vi "LvJDS2900_Sub_Inquiry.vi"(8 "error in (no error)":errorcluster caption="エラー入力（エラーなし）", 10 "Command":string, 11 "VISA rsrc":refnum<visa-resource-name>) -> (0 "error out":errorcluster caption="エラー出力", 1 "Response":string, 3 "VISA rsrc out":refnum<visa-resource-name>)   [LabVIEW 2014]
panel:
  # ":r<nn>=<x>"
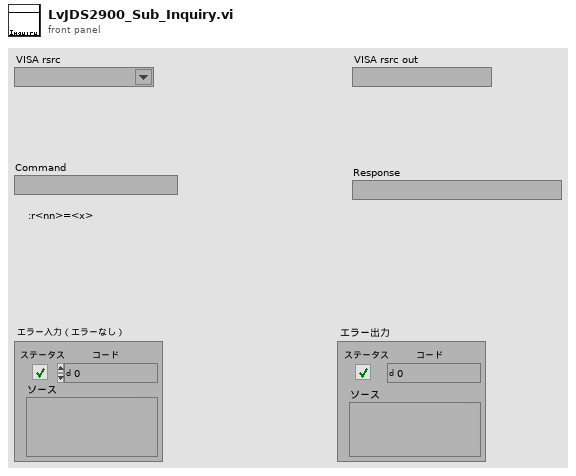
[diagram p1: front panel]
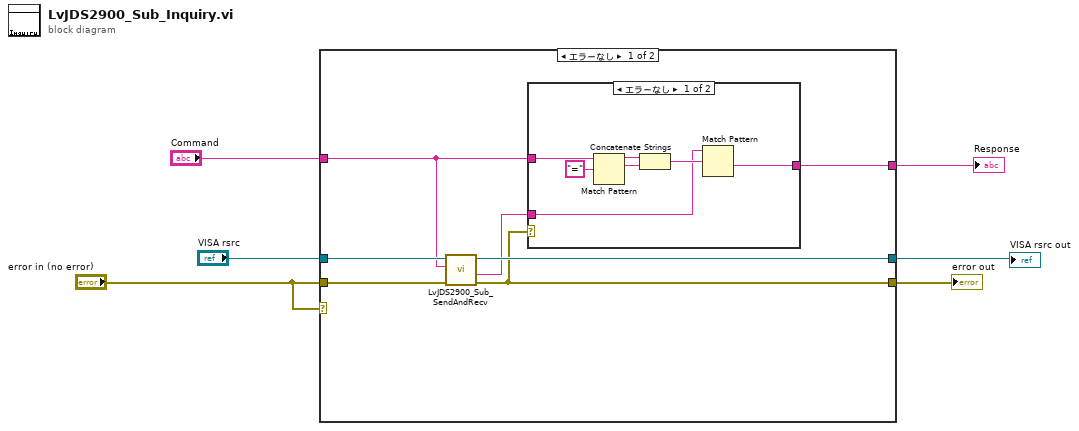
[diagram p0: block diagram]
diagram:
  n1 = case shown="エラーなし" "error in (no error)" {
    tunnel: "VISA rsrc" -> [w13 w21]
    tunnel: "Command" -> [w10 _]
    tunnel: [w9 w22] -> w4
    tunnel: "error in (no error)" -> [w11 w22]
    tunnel: [w12 w21] -> w3
    tunnel: [w7 _] -> w1
    frame No Error {
      n2 = call "LvJDS2900_Sub_SendAndRecv.vi"("error in (no error)"=w11, "Command"=w10, "VISA rsrc"=w13) -> ("error out"=w9:errorcluster, "Response"=w8:string, "VISA rsrc out"=w12:refnum<visa-resource-name>)  [unwired: 6 in]
      n3 = case shown="エラーなし" w9 {
        tunnel: w10 -> [w19 _]
        tunnel: w8 -> [w15 _]
        tunnel: [w14 _] -> w7
        frame No Error {
          n4 = Match Pattern(string=w19, regular expression="=" ("正規表現")) -> (before substring=w18:string, match substring=w17:string)  [unwired: 1 in, 2 out]
          n5 = Concatenate Strings(w18, w17) -> (w16:string)
          n6 = Match Pattern(string=w15, regular expression=w16) -> (after substring=w14:string)  [unwired: 1 in, 3 out]
        }
        frame Error {
        }
      }
    }
    frame Error {
    }
  }
  "error out" <- w4
  "VISA rsrc out" <- w3
  "Response" <- w1
